vi "ConvertTachSignalToPulses.vi"(8 "error in (no error)":errorcluster, 10 "tachometer signal":waveform(dbl), 11 "duration":dbl=213.0 format="%#_13g") -> (0 "error out":errorcluster, 1 "tachometer pulses U32":cluster{"Data":u32[]}[](array[cluster]), 2 "Tachometer Pulses":T1[](array[typedef]), 3 "duration out":dbl)   [LabVIEW 2017]
uses:
  <vilib>/addons/InsightCM/Utilities/Analysis/Shared/controls/PulsePositions.ctl
  <vilib>/addons/InsightCM/Devices/Shared/Cms/CmsAcquisition/CmsAcquisition.lvlib
  <vilib>/addons/InsightCM/Utilities/Analysis/Shared/AnalysisHelper.lvlib
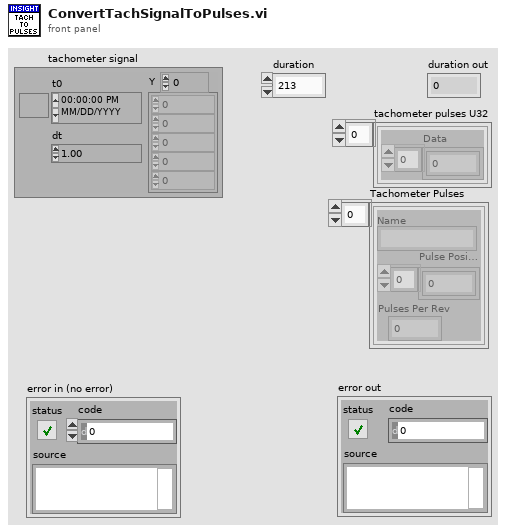
[diagram p1: front panel]
types:
  T1 = typedef "AnalysisHelper.lvlib/PulsePositions.ctl" = cluster{"Name":string, "Pulse Position Data":dbl[], "Pulses Per Rev":i32}
  T2 = typedef "rolloverState.ctl" = cluster{"prev value":u32, "total add":dbl}
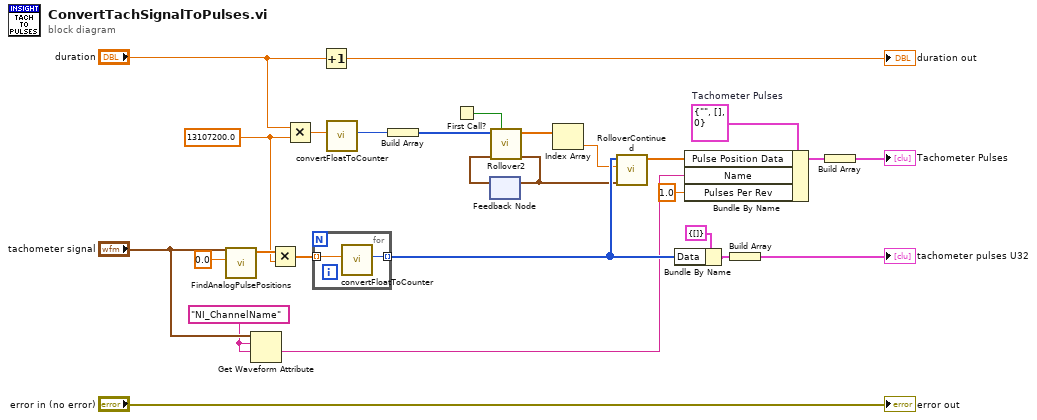
[diagram p0: block diagram]
diagram:
  w3 = "NI_ChannelName"
  w7 = T1 {"Name"="", "Pulse Position Data"=[], "Pulses Per Rev"=0}  # Tachometer Pulses
  w13 = 13107200.0
  n1 = call <vilib>:"FindAnalogPulsePositions.vi"("level"=0.0 ("Level"), "tach signal"="tachometer signal") -> ("pulse positions"=w25:dbl[])  [unwired: 9 in]
  n2 = Get Waveform Attribute(5:w3, 6:w3, 7:"tachometer signal") -> (1:w4:string)  [unwired: 1 in, 3 out]
  n3 = Multiply(x=w25, y=w13) -> (x*y=w22:dbl[])
  n4 = Multiply(x="duration", y=w13) -> (x*y=w14:dbl)
  n5 = for {
    tunnel: w22 -> [w29] mode=indexing
    tunnel: [w28] -> w19 mode=indexing
    n6 = call <vilib>:"convertFloatToCounter.vi"("Numeric"=w29) -> ("Counter Version"=w28:u32)  [unwired: 10 in]
  }
  n7 = Increment(x="duration") -> (x+1=→"duration out":dbl)
  n8 = call <vilib>:"convertFloatToCounter.vi"("Numeric"=w14) -> ("Counter Version"=w12:u32)  [unwired: 10 in]
  n9 = Build Array(w12) -> (w11:u32[])
  n10 = First Call?() -> (First Call?: T/F=w21:bool)
  n11 = feedback #1() -> (w20:T2)  [unwired: 1 in]
  n12 = call <vilib>:"Rollover2.vi"("reset"=w21, "rollover state"=w20, "counter"=w11) -> ("rollover state"=w18:T2, "counter"=w17:dbl[])  [unwired: 7 in]
  n13 = feedback-in #1(w18) -> ()
  n14 = Index Array(array=w17) -> (element=w15:dbl)  [unwired: 1 in]
  n15 = call <vilib>:"RolloverContinued.vi"("rollover state"=w18, "OSClkStart"=w15, "counter"=w19) -> ("this block"=w16:dbl[])  [unwired: 5 in, 3 out]
  n16 = Bundle By Name(cluster=cluster{"Data":u32[]} {"Data"=[]} ("PulsePositions"), "Data"=w19) -> (w24:cluster{"Data":u32[]})
  n17 = Bundle By Name(cluster=w7, "Pulse Position Data"=w16, "Name"=w4, "Pulses Per Rev"=1.0) -> (w26:T1)
  n18 = Build Array(w24) -> (→"tachometer pulses U32":cluster{"Data":u32[]}[])
  n19 = Build Array(w26) -> (→"Tachometer Pulses":T1[])
  "error out" <- "error in (no error)"
